vi "Stop Measuring.vi"(8 "error in (no error)":errorcluster, 11 "Coverage Analyzer in":refnum<class "Coverage Analyzer.lvclass">) -> (0 "error out":errorcluster, 3 "Coverage Analyzer out":refnum<class "Coverage Analyzer.lvclass">)   [LabVIEW 2020, in "Coverage Analyzer.lvlib" / "Coverage Analyzer.lvclass"]
uses:
  Coverage Analyzer.lvclass
  Coverage Analyzer.lvclass/Coverage Analyzer.ctl
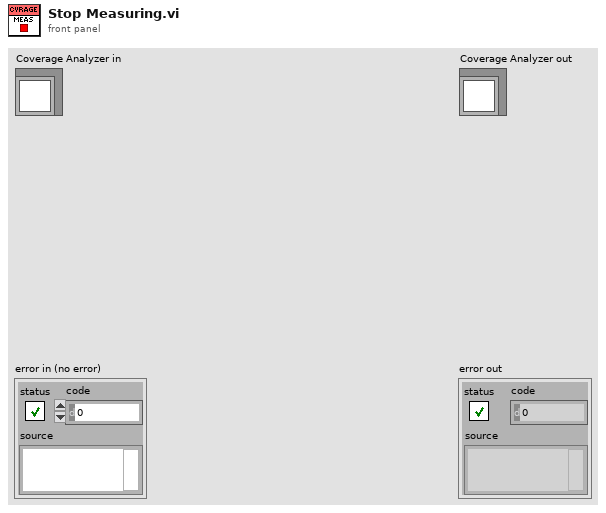
[diagram p1: front panel]
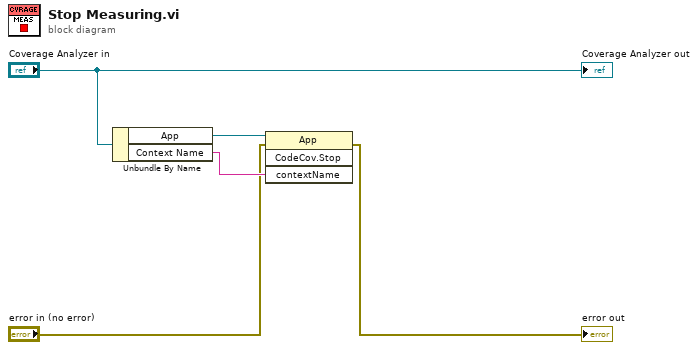
[diagram p0: block diagram]
diagram:
  n1 = Unbundle By Name("Coverage Analyzer in") -> ("App"=w4:refnum<vi>, "Context Name"=w3:string)
  n2 = invoke class="App" method="CodeCov.Stop"(reference=w4, error in="error in (no error)", "contextName"=w3) -> (error out=→"error out":errorcluster)  [unwired: 1 in, 3 out]
  "Coverage Analyzer out" <- "Coverage Analyzer in"
